vi "Constructor.vi"(8 "error in (no error)":errorcluster) -> (0 "error out":errorcluster, 3 "Block Diagram":refnum<class "VI.lvclass">)   [LabVIEW 2015, in "VI.lvclass"]
uses:
  VI.lvclass
  Main Sequence/Main Sequence.lvclass
  DMA Loop/DMA Loop.lvclass
  VI.lvclass/VI.ctl
  Module Loop/Module Loop.lvclass
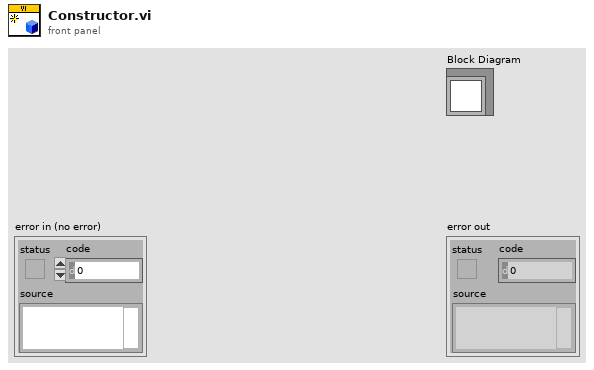
[diagram p1: front panel]
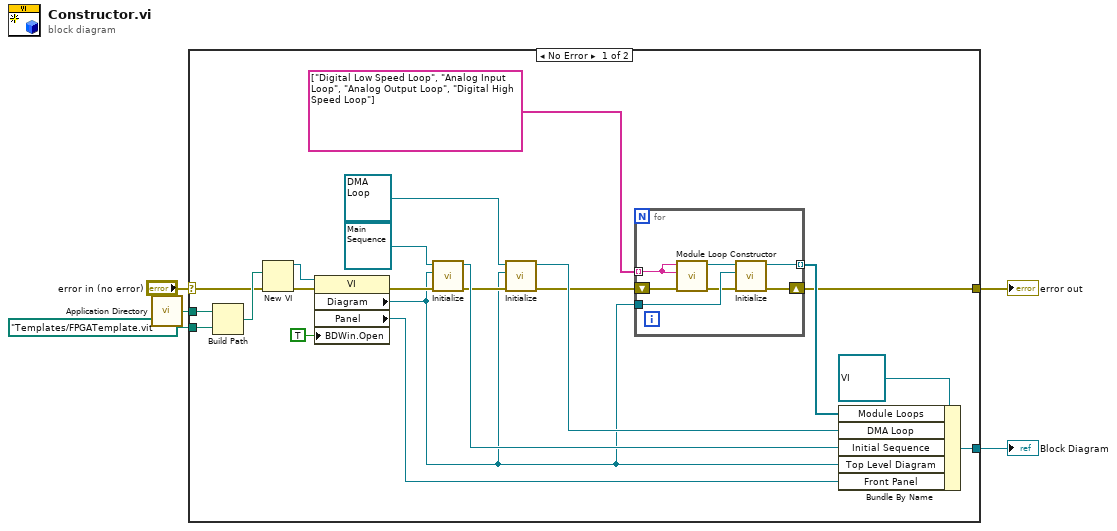
[diagram p0: block diagram]
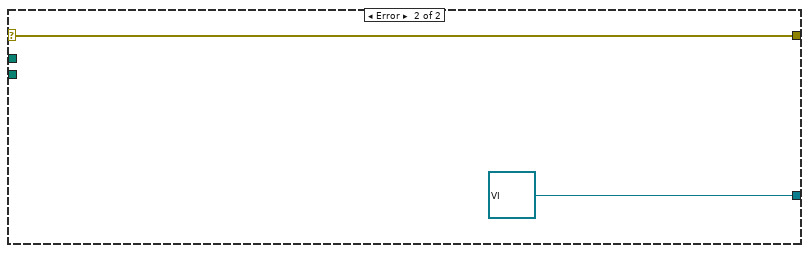
[diagram p2: hidden frame]
diagram:
  n1 = call <vilib>:"Application Directory.vi"() -> ("Application Directory"=w3:path)
  n2 = case shown="No Error" "error in (no error)" {
    selector: "error in (no error)" -> [w8 w35]
    tunnel: [w22 refnum<class "VI.lvclass"> refnum ("Block Diagram.lvclass")] -> w5
    tunnel: [w19 w35] -> w4
    tunnel: w3 -> [w17 _]
    tunnel: path "Templates/FPGATemplate.vit" ("Application Directory") -> [w16 _]
    frame No Error {
      n3 = Build Path(base path=w17, name or relative path=w16) -> (appended path=w15:path)
      n4 = New VI(8:w8, 10:w15) -> (0:w13:errorcluster, 3:w14:refnum<vi>)  [unwired: 5 in]
      n5 = property class="VI"(reference=w14, error in=w13, "BDWin.Open"=TRUE ("Block Diagram Window:Open")) -> (error out=w12:errorcluster, "Diagram"=w11:refnum<vi>, "Panel"=w9:refnum<vi>)  [unwired: 1 out]
      n6 = call-dynamic "Initialize.vi"("error in (no error)"=w12, "Top Level Diagram"=w11, "Initial Sequence in"=refnum<class "Main Sequence.lvclass"> refnum ("Initial Sequence.lvclass")) -> ("error out"=w23:errorcluster, "Initial Sequence out"=w24:refnum<class "Main Sequence.lvclass">)  [unwired: 7 in]
      n7 = call-dynamic "Initialize.vi"("error in (no error)"=w23, "Top Level Diagram"=w11, "DMA Loop in"=refnum<class "DMA Loop.lvclass"> refnum ("DMA Loop.lvclass")) -> ("error out"=w20:errorcluster, "DMA Loop out"=w25:refnum<class "DMA Loop.lvclass">)  [unwired: 7 in]
      n8 = for {
        tunnel: w11 -> [w32]
        shift-right: [w33] -> w19
        shift-left: w20 -> [w29]
        tunnel: [w31] -> w21 mode=indexing
        tunnel: string[] ["Digital Low Speed Loop", "Analog Input Loop", "Analog Output Loop", "Digital High Speed Loop"] -> [w27] mode=indexing
        n9 = call "Module Loop Constructor.vi"("error in (no error)"=w29, "Name"=w27, "Type"=w27) -> ("error out"=w28:errorcluster, "Module Loop.lvclass"=w30:refnum<class "Module Loop.lvclass">)  [unwired: 7 in]
        n10 = call-dynamic "Initialize.vi"("error in (no error)"=w28, "Top Level Diagram"=w32, "IO Loop in"=w30) -> ("error out"=w33:errorcluster, "IO Loop out"=w31:refnum<class "Module Loop.lvclass">)  [unwired: 7 in]
      }
      n11 = Bundle By Name(cluster=refnum<class "VI.lvclass"> refnum ("Block Diagram.lvclass"), "Module Loops"=w21, "DMA Loop"=w25, "Initial Sequence"=w24, "Top Level Diagram"=w11, "Front Panel"=w9) -> (w22:refnum<class "VI.lvclass">)
    }
    frame Error {
    }
  }
  "Block Diagram" <- w5
  "error out" <- w4
